vi "publish -- get frequency and voltage -- test.vi"() -> ()   [LabVIEW 2017]
uses:
  publisher action.ctl
panel:
  out "gamma OUT (Hz)":dbl=1000.0
  out "Voltage out (V)":cdb=1.133070214302279+0.0i
  out "freq out (Hz)":dbl=1000.0 format="%#_10f"
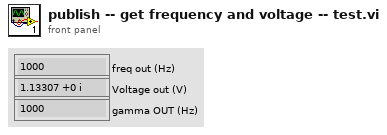
[diagram p1: front panel]
types:
  T1 = typedef "publisher action.ctl" = enum16{"set", "get"}
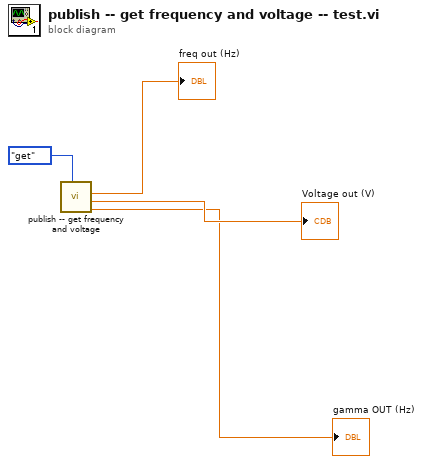
[diagram p0: block diagram]
diagram:
  n1 = call "publish -- get frequency and voltage.vi"("publisher action"=publisher_action."get") -> ("gamma OUT (Hz)"=→"gamma OUT (Hz)":dbl, "Voltage out (V)"=→"Voltage out (V)":cdb, "freq out (Hz)"=→"freq out (Hz)":dbl)  [unwired: 8 in]
